vi "SCPI Configure Program Values.vi"(6 "Step":u16, 7 "Elapse Time":u16, 8 "error in (no error)":errorcluster, 9 "Set Current":dbl format="%.2g", 10 "Set Voltage":dbl format="%.1g", 11 "VISA resource name":refnum<visa-resource-name>) -> (0 "error out":errorcluster, 3 "VISA resource name out":refnum<visa-resource-name>)   [LabVIEW 2021, in "BK Precision 169XB.lvlib"]
doc: "Configures over current protection (OCP). Specify the output current limit value and the behavior of the power supply when the output current is greater than or equal to that value."
uses:
  BK Precision 169XB.lvlib
panel:
  in  "MIN":dbl format="%.1g"
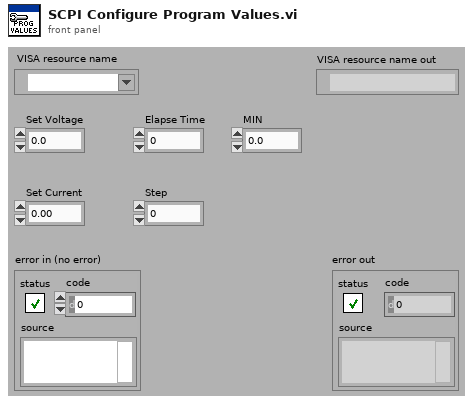
[diagram p1: front panel]
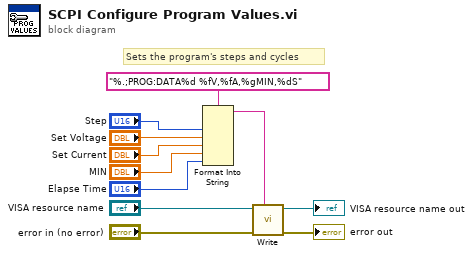
[diagram p0: block diagram]
diagram:
  # "Sets the program's steps and cycles"
  n1 = Format Into String(format string="%.;PROG:DATA%d %fV,%fA,%gMIN,%dS", "Step", "Set Voltage", "Set Current", "MIN", "Elapse Time") -> (resulting string=w11:string)  [unwired: 2 in, 1 out]
  n2 = call "Write.vi"("Input String"=w11, "error in (no error)"="error in (no error)", "VISA resource name"="VISA resource name") -> ("error out"=→"error out":errorcluster, "VISA resource name out"=→"VISA resource name out":refnum<visa-resource-name>)  [unwired: 6 in, 1 out]
